vi "acknowledgeIRQ.vi"(8 "error in (no error)":errorcluster, 10 "IRQs":i32[](array[numeric]), 11 "Modbus in":refnum<class "Modbus.lvclass">) -> (0 "error out":errorcluster, 3 "Modbus out":refnum<class "Modbus.lvclass">)   [LabVIEW 2016, in "RTModbus.lvlib" / "Modbus.lvclass"]
uses:
  Modbus.lvclass
  Modbus.lvclass/Modbus.ctl
  Common_RT_FPGA/IIRQ/IIRQ.lvclass
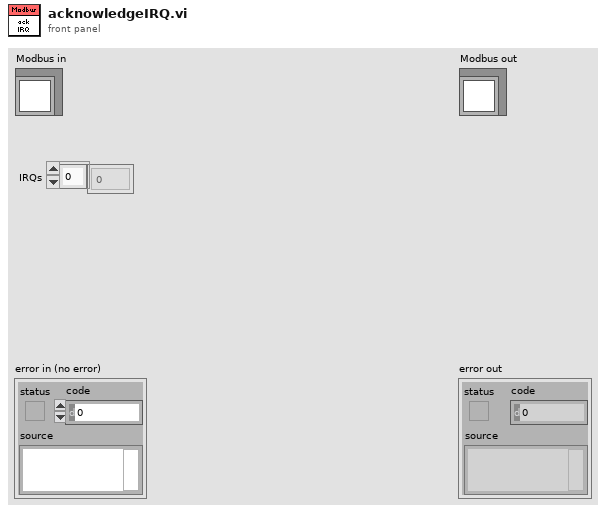
[diagram p1: front panel]
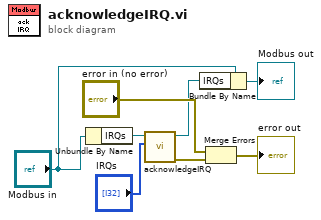
[diagram p0: block diagram]
diagram:
  n1 = Unbundle By Name("Modbus in") -> ("IRQs"=w5:refnum<class "IIRQ.lvclass">)
  n2 = call-dynamic "acknowledgeIRQ.vi"("IRQs"="IRQs", "IIRQ in"=w5) -> ("error out"=w1:errorcluster, "IIRQ out"=w3:refnum<class "IIRQ.lvclass">)  [unwired: 8 in]
  n3 = Bundle By Name(cluster="Modbus in", "IRQs"=w3) -> (→"Modbus out":refnum<class "Modbus.lvclass">)
  n4 = Merge Errors("error in (no error)", w1) -> (→"error out":errorcluster)
